vi "read_class.vi"(8 "error in (no error)":errorcluster) -> (0 "error out":errorcluster, 3 "class out":refnum<class "v1.lvclass">)   [LabVIEW 2015, in "lv-dialog.lvlib" / "v1.lvlib"]
uses:
  v1.lvlib
  class/v1.lvclass
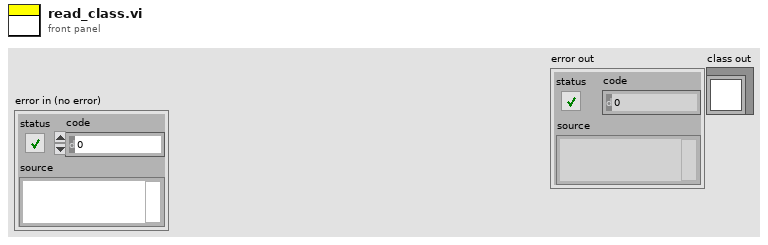
[diagram p1: front panel]
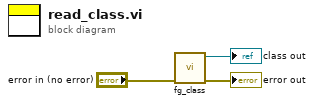
[diagram p0: block diagram]
diagram:
  n1 = call "fg_class.vi"("error in (no error)"="error in (no error)") -> ("error out"=→"error out":errorcluster, "class out"=→"class out":refnum<class "v1.lvclass">)  [unwired: 9 in]
